vi "Iterate.vi"(10 "Iteration Attempts":u16, 11 "Start Value":cdb) -> (1 "Iteration Value":cdb, 2 "Escaped?":bool, 3 "Iteration":u16)   [LabVIEW 2016]
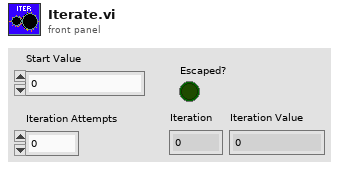
[diagram p1: front panel]
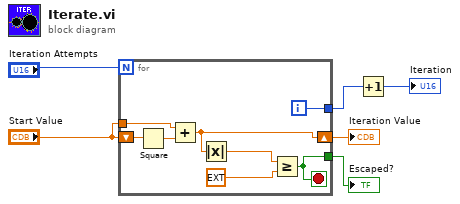
[diagram p0: block diagram]
diagram:
  n1 = for {
    N: "Iteration Attempts" -> [_]
    shift-right: [w11] -> w1
    shift-left: "Start Value" -> [w14]
    tunnel: "Start Value" -> [w12]
    tunnel: [w9] -> w5
    tunnel: [w8] -> w4
    i -> [w9]
    stop <- w8 stop-if-true
    n2 = Square(x=w14) -> (x^2=w13:cdb)
    n3 = Add(x=w12, y=w13) -> (x+y=w11:cdb)
    n4 = Absolute Value(x=w11) -> (abs(x)=w7:dbl)
    n5 = Greater Or Equal?(x=w7, y=ext 2.0) -> (x >= y?=w8:bool)
  }
  "Escaped?" <- w4
  "Iteration Value" <- w1
  n6 = Increment(x=w5) -> (x+1=→"Iteration":i32)
